vi "Get Sensor Signals.vi"(7 "Filter Cluster":string="RDB_SENSOR_STATE", 8 "error in (no error)":errorcluster, 11 "Item Ref in":T1 format="%.0x") -> (0 "error out (no error)":errorcluster, 1 "Sensor Signals":string[](array[string]), 2 "Sensor Names":string[](array[string]), 3 "Item Ref out":T1 format="%.0x")   [LabVIEW 2020, in "Vires VTD System Explorer.lvlib"]
uses:
  Vires VTD System Explorer.lvlib
  <vilib>/NI VeriStand/Custom Device API/Custom Device Item Ref.ctl
  <vilib>/xnet/xnet.llb/XNET String To IO Name (Database Alias).vi
  <resource>/objmgr/xnet.rc
  <vilib>/NI VeriStand/Custom Device API/Custom Device API.lvlib
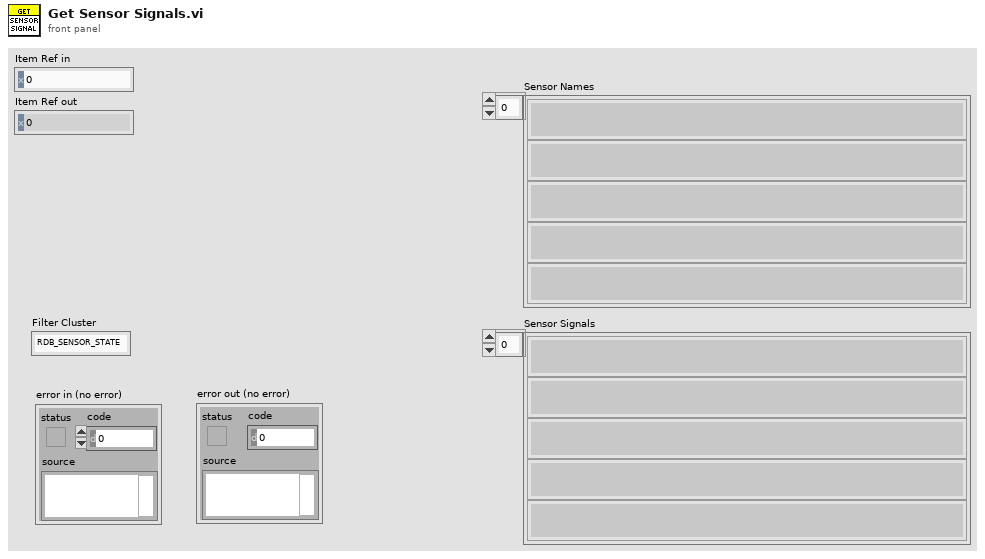
[diagram p1: front panel]
types:
  T1 = typedef "Custom Device API.lvlib/Custom Device Item Ref.ctl" = u64
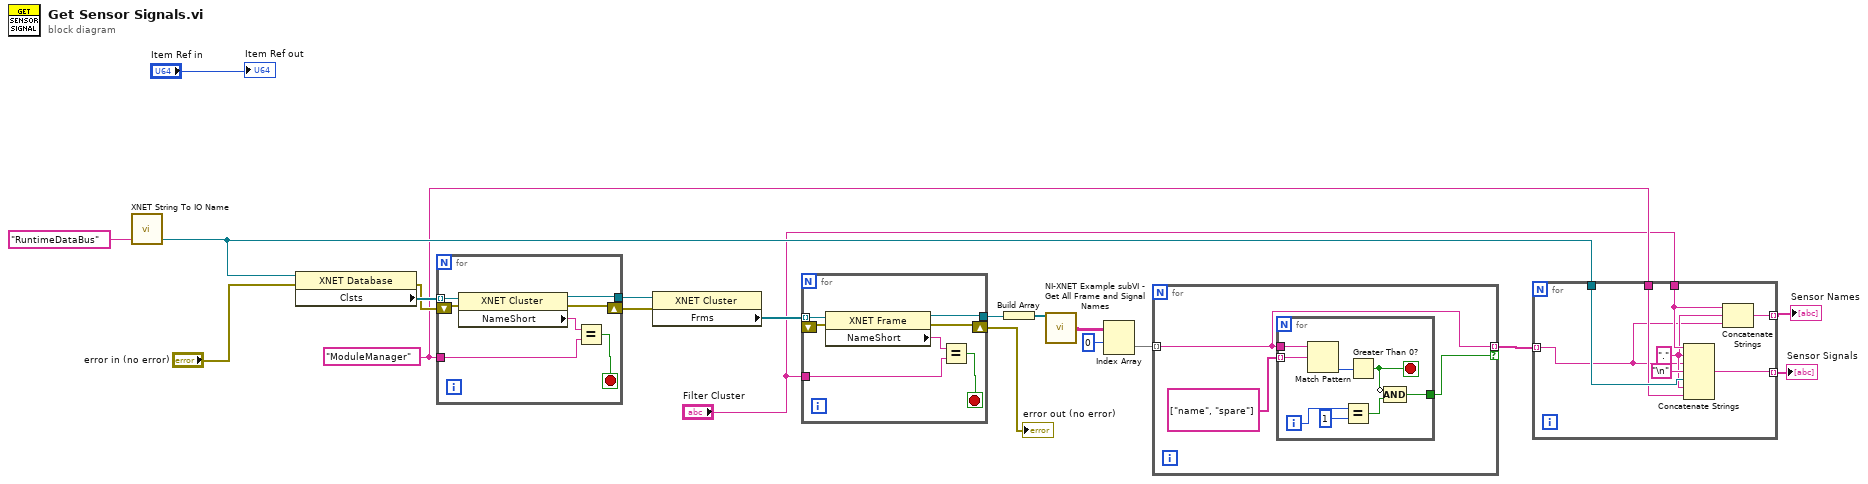
[diagram p0: block diagram]
diagram:
  w7 = "ModuleManager" ("Filter Cluster")
  n1 = call-poly <vilib>:"XNET String To IO Name.vi"("string"="RuntimeDataBus" ("element")) -> ("XNET Database"=w8:refnum<k21>)  [unwired: 4 out]
  n2 = property class="XNET Database"(reference=w8, error in="error in (no error)") -> (error out=w18:errorcluster, "Clsts"=w19:refnum<k21>[])  [unwired: 1 out]
  n3 = for {
    tunnel: w19 -> [w27] mode=indexing
    tunnel: [w26] -> w17
    shift-right: [w22] -> w16
    shift-left: w18 -> [w23]
    tunnel: w7 -> [w21]
    stop <- w25 stop-if-true
    n4 = property class="XNET Cluster"(reference=w27, error in=w23) -> (reference out=w26:refnum<k21>, error out=w22:errorcluster, "NameShort"=w24:string)
    n5 = Equal?(x=w24, y=w21) -> (x = y?=w25:bool)
  }
  n6 = property class="XNET Cluster"(reference=w17, error in=w16) -> ("Frms"=w15:refnum<k21>[])  [unwired: 2 out]
  n7 = for {
    tunnel: w15 -> [w34] mode=indexing
    tunnel: [w33] -> w14
    shift-right: [w29] -> w2
    shift-left: _ -> [w30]
    tunnel: "Filter Cluster" -> [w28]
    stop <- w32 stop-if-true
    n8 = property class="XNET Frame"(reference=w34, error in=w30) -> (reference out=w33:refnum<k21>, error out=w29:errorcluster, "NameShort"=w31:string)
    n9 = Equal?(x=w31, y=w28) -> (x = y?=w32:bool)
  }
  "error out (no error)" <- w2
  n10 = Build Array(w14) -> (w13:refnum<k21>[])
  n11 = call "NI-XNET Example subVI - Get All Frame and Signal Names.vi"("XNET Frames"=w13) -> ("Signal Names"=w11:string[][])  [unwired: 10 in, 4 out]
  n12 = Index Array(array=w11, index (row)=0) -> (element=w10:string[])  [unwired: 1 in]
  n13 = for {
    tunnel: w10 -> [w36] mode=indexing
    tunnel: [w36] -> w9 mode=indexing if=w35
    n14 = for {
      tunnel: string[] ["name", "spare"] -> [w45] mode=indexing
      tunnel: w36 -> [w44]
      tunnel: [w38] -> w35
      i -> [w43]
      stop <- w39 stop-if-true
      n15 = Match Pattern(string=w44, regular expression=w45) -> (offset past match=w41:i32)  [unwired: 1 in, 3 out]
      n16 = Equal?(x=w43, y=1) -> (x = y?=w40:bool)
      n17 = Greater Than 0?(x=w41) -> (x > 0?=w39:bool)
      n18 = Compound Arithmetic op=AND(invert w39, w40) -> (w38:bool)
    }
  }
  n19 = for {
    tunnel: w9 -> [w47] mode=indexing
    tunnel: "Filter Cluster" -> [w49]
    tunnel: w8 -> [w52]
    tunnel: w7 -> [w51]
    tunnel: [w50] -> w6 mode=indexing
    tunnel: [w46] -> w4 mode=indexing
    w48 = "." ("string")
    n20 = Concatenate Strings(w49, w48, w47, "\n", w52, w48, w51) -> (w50:string)
    n21 = Concatenate Strings(w49, w48, w47) -> (w46:string)
  }
  "Sensor Signals" <- w6
  "Sensor Names" <- w4
  "Item Ref out" <- "Item Ref in"
